vi "poly_notify_boolean_notifier_name.vi"(2 "notifier name":string) -> (7 "notified?":bool)   [LabVIEW 2015]
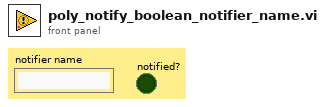
[diagram p1: front panel]
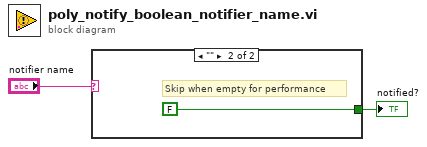
[diagram p0: block diagram]
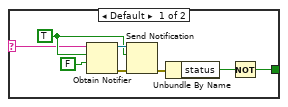
[diagram p2: hidden frame]
diagram:
  n1 = case shown="\"\"" "notifier name" {
    selector: "notifier name" -> [w3 _]
    tunnel: [w8 FALSE] -> w2
    frame Default {
      w6 = TRUE
      n2 = Obtain Notifier(name (unnamed)=w3, notification data type=w6, create if not found? (T)=FALSE) -> (notifier out=w7:refnum<notifier>, error out=w4:errorcluster)  [unwired: 1 in, 1 out]
      n3 = Send Notification(notification=w6, notifier=w7, error in (no error)=w4) -> (error out=w10:errorcluster)  [unwired: 1 out]
      n4 = Unbundle By Name(w10) -> ("status"=w9:bool)
      n5 = Not(x=w9) -> (.not. x?=w8:bool)
    }
    frame "" {
      # "Skip when empty for performance"
    }
  }
  "notified?" <- w2
